vi "Generator.vi"() -> ()   [LabVIEW 2015]
uses:
  Components/YAML Parser Class/Add Attribute - String.vi
  Components/YAML Parser Class/Add Attribute - DBL.vi
  Components/YAML Parser Class/Add Attribute - Datetime.vi
  Components/YAML Parser Class/Add Attribute - Timestamp.vi
  Components/YAML Parser Class/Add Attribute - Array String.vi
  Components/YAML Parser Class/Add Attribute - Object.vi
  Components/YAML Parser Class/Add Attribute - Null.vi
  Components/YAML Parser Class/Add Attribute - Class.vi
  Components/YAML Parser Class/Add Attribute - Refnum.vi
  Components/YAML Parser Class/Add Attribute - Analog Waveform.vi
  Components/YAML Parser Class/Flush.vi
  Components/YAML Parser Class/YAML Parser.lvclass
  <vilib>/measure/NI_MABase.lvlib
panel:
  in  "YAML Tree":string(tree)
  out "error out":errorcluster
  out "YAML String":string
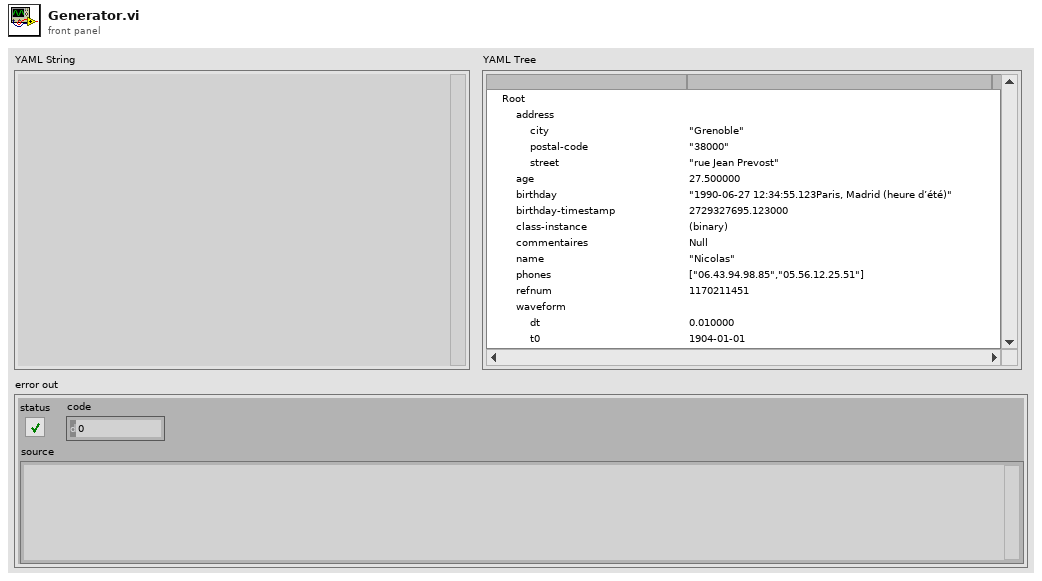
[diagram p1: front panel]
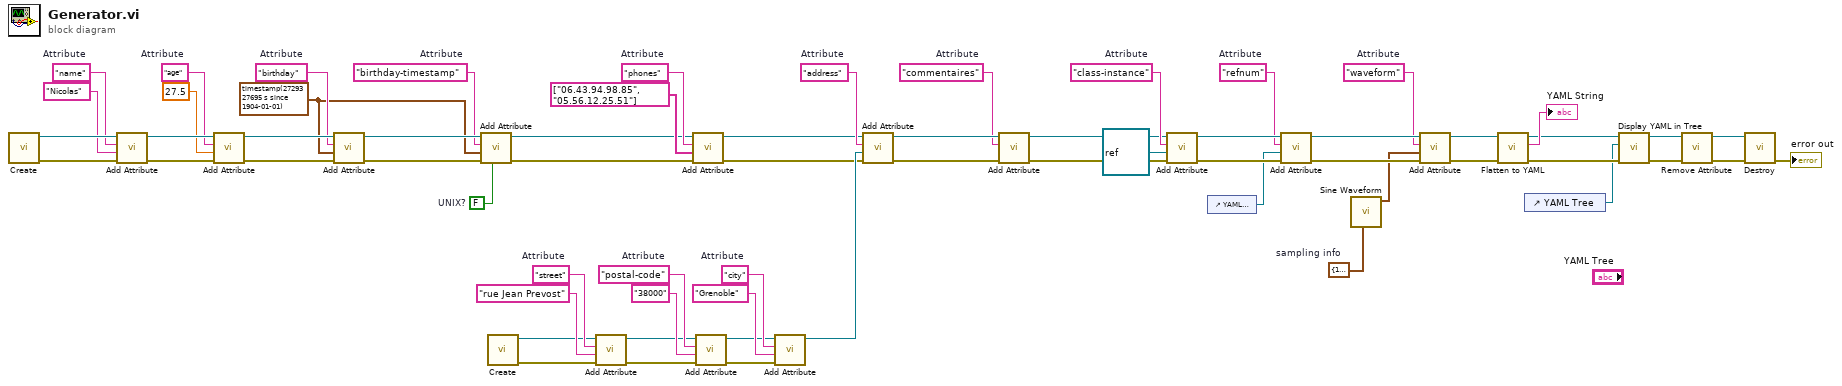
[diagram p0: block diagram]
diagram:
  w1 = "commentaires"  # Attribute
  w7 = cluster{"Fs":dbl, "#s":dbl} {"Fs"=100.0, "#s"=10.0}  # sampling info
  w9 = "waveform"  # Attribute
  w10 = "refnum"  # Attribute
  w17 = FALSE  # UNIX?
  w19 = timestamp(2729327695.123 s since 1904-01-01) ("Value")
  w23 = "birthday-timestamp"  # Attribute
  w20 = "birthday"  # Attribute
  w24 = "class-instance"  # Attribute
  w37 = "phones"  # Attribute
  w41 = "address"  # Attribute
  w46 = "city"  # Attribute
  w49 = "postal-code"  # Attribute
  w52 = "street"  # Attribute
  w55 = "age"  # Attribute
  w61 = "name"  # Attribute
  n1 = call "Create.vi"() -> ("error out"=w62:errorcluster, "YAML Parser out"=w63:refnum<class "YAML Parser.lvclass">)  [unwired: 10 in]
  n2 = call-poly "Add Attribute.vi"("error in (no error)"=w62, "Value"="Nicolas", "Attribute"=w61, "YAML Parser in"=w63) -> ("error out"=w56:errorcluster, "YAML Parser out"=w57:refnum<class "YAML Parser.lvclass">)  [unwired: 6 in]
  n3 = call-poly "Add Attribute.vi"("error in (no error)"=w56, "Value"=27.5, "Attribute"=w55, "YAML Parser in"=w57) -> ("error out"=w27:errorcluster, "YAML Parser out"=w28:refnum<class "YAML Parser.lvclass">)  [unwired: 5 in, 1 out]
  n4 = call-poly "Add Attribute.vi"("error in (no error)"=w27, "Value"=w19, "Attribute"=w20, "YAML Parser in"=w28) -> ("error out"=w25:errorcluster, "YAML Parser out"=w26:refnum<class "YAML Parser.lvclass">)  [unwired: 6 in]
  n5 = call-poly "Add Attribute.vi"("UNIX?"=w17, "error in (no error)"=w25, "Value"=w19, "Attribute"=w23, "YAML Parser in"=w26) -> ("error out"=w21:errorcluster, "YAML Parser out"=w22:refnum<class "YAML Parser.lvclass">)  [unwired: 5 in]
  n6 = call "Create.vi"() -> ("error out"=w51:errorcluster, "YAML Parser out"=w50:refnum<class "YAML Parser.lvclass">)  [unwired: 10 in]
  n7 = call-poly "Add Attribute.vi"("error in (no error)"=w51, "Value"="rue Jean Prevost", "Attribute"=w52, "YAML Parser in"=w50) -> ("error out"=w44:errorcluster, "YAML Parser out"=w45:refnum<class "YAML Parser.lvclass">)  [unwired: 6 in]
  n8 = call-poly "Add Attribute.vi"("error in (no error)"=w21, "Value"=string[] ["06.43.94.98.85", "05.56.12.25.51"], "Attribute"=w37, "YAML Parser in"=w22) -> ("error out"=w38:errorcluster, "YAML Parser out"=w39:refnum<class "YAML Parser.lvclass">)  [unwired: 6 in]
  n9 = call-poly "Add Attribute.vi"("error in (no error)"=w44, "Value"="38000", "Attribute"=w49, "YAML Parser in"=w45) -> ("error out"=w42:errorcluster, "YAML Parser out"=w43:refnum<class "YAML Parser.lvclass">)  [unwired: 6 in]
  n10 = call-poly "Add Attribute.vi"("error in (no error)"=w42, "Value"="Grenoble", "Attribute"=w46, "YAML Parser in"=w43) -> ("YAML Parser out"=w40:refnum<class "YAML Parser.lvclass">)  [unwired: 6 in, 1 out]
  n11 = call-poly "Add Attribute.vi"("error in (no error)"=w38, "Value"=w40, "Attribute"=w41, "YAML Parser in"=w39) -> ("error out"=w2:errorcluster, "YAML Parser out"=w3:refnum<class "YAML Parser.lvclass">)  [unwired: 6 in]
  n12 = call-poly "Add Attribute.vi"("error in (no error)"=w2, "Attribute"=w1, "YAML Parser in"=w3) -> ("error out"=w4:errorcluster, "YAML Parser out"=w5:refnum<class "YAML Parser.lvclass">)  [unwired: 7 in]
  n13 = call-poly "Add Attribute.vi"("error in (no error)"=w4, "Value"=refnum<class> refnum ("LabVIEW Object"), "Attribute"=w24, "YAML Parser in"=w5) -> ("error out"=w15:errorcluster, "YAML Parser out"=w16:refnum<class "YAML Parser.lvclass">)  [unwired: 6 in]
  n14 = control-ref of="YAML String"() -> (w6:refnum<vi>)
  n15 = call-poly "Add Attribute.vi"("error in (no error)"=w15, "Value"=w6, "Attribute"=w10, "YAML Parser in"=w16) -> ("error out"=w13:errorcluster, "YAML Parser out"=w14:refnum<class "YAML Parser.lvclass">)  [unwired: 6 in]
  n16 = call <vilib>:"Sine Waveform.vi"("sampling info"=w7) -> ("signal out"=w8:waveform(dbl))  [unwired: 9 in, 1 out]
  n17 = call-poly "Add Attribute.vi"("error in (no error)"=w13, "Value"=w8, "Attribute"=w9, "YAML Parser in"=w14) -> ("error out"=w11:errorcluster, "YAML Parser out"=w12:refnum<class "YAML Parser.lvclass">)  [unwired: 6 in]
  n18 = call "Flatten to YAML.vi"("error in (no error)"=w11, "YAML Parser in"=w12) -> ("error out"=w34:errorcluster, "YAML String"=→"YAML String":string, "YAML Parser out"=w35:refnum<class "YAML Parser.lvclass">)  [unwired: 7 in]
  n19 = control-ref of="YAML Tree"() -> (w33:refnum<vi>)
  n20 = call "Display YAML in Tree.vi"("error in (no error)"=w34, "Tree Refnum"=w33, "YAML Parser in"=w35) -> ("error out"=w31:errorcluster, "YAML Parser out"=w32:refnum<class "YAML Parser.lvclass">)  [unwired: 7 in]
  n21 = call-poly "Remove Attribute.vi"("error in (no error)"=w31, "YAML Parser in"=w32) -> ("error out"=w30:errorcluster, "YAML Parser out"=w29:refnum<class "YAML Parser.lvclass">)  [unwired: 8 in]
  n22 = call "Destroy.vi"("error in (no error)"=w30, "YAML Parser in"=w29) -> ("error out"=→"error out":errorcluster)  [unwired: 9 in]
